vi "SVFA Real and Imaginary to Magnitude and Phase (1 Ch).vi"(0 "real spectrum":cluster{"x0":dbl, "dx":dbl, "real part":dbl[]}, 2 "imaginary spectrum":T8, 4 "spectrum info in":T2={"channel name"="", "description"="", "x-axis units"=0, "spectral info"={"spectrum type"=enum."Power [Magnitude^2]", "linear/dB"=enum."linear", "window"=0, "window size"=0, "FFT size"=0}, "engineering units"=0, "custom label"="", "dB reference [EU]"=0.0, "peak units"=enum."rms", "weighting filter"=0, "spectral density?"=FALSE, "unit label"="", "spectrum skewed?"=FALSE, "complimentary spectrum units"=enum."none"} {"x-axis units" items=["Time (s)"=0, "Frequency-CB (Hz)"=1, "Frequency-CPB (Hz)"=1248, "Frequency-Arbitrary (Hz)"=2357, "Quefrency (s)"=2, "Revolutions (rev)"=3, "Order"=4, "Speed (RPM)"=11, "Speed (rad/s)"=21, "Index"=65535]; "weighting filter" items=["Linear", "A-weighting", "B-weighting", "C-weighting", "ITU-R 468-4", "Dolby", "CCITT", "C-message", "Wb", "Wc", "Wd", "We", "Wf", "Wh", "Wj", "Wk", "Wm", "AES17 20 kHz lowpass", "AES17 40 kHz lowpass", "AES17 20 kHz highpass", "AES17 40 kHz highpass"]; "dB reference [EU]" format="%.2f"; "engineering units" items=["custom..."=0, "V"=1, "A"=21, "C"=30, "pC"=31, "s"=32, "-"=29, "Pa"=2, "N"=20, "g"=3, "m/s^2"=4, "m/s"=5, "m"=6, "mm/s"=12, "mm"=13, "micron/s"=14, "micron"=15, "in/s^2"=7, "in/s"=8, "in"=9, "mil/s"=10, "mil"=11, "rad/s^2"=16, "rad/s"=17, "rad"=18, "deg/s^2"=26, "deg/s"=27, "deg"=28, "RPM"=22, "cycle/s^2"=23, "Hz"=24, "cycle"=25, "strain"=19]; "spectral info"."window" items=["None "=0, "Hanning"=1, "Hamming"=2, "Blackman-Harris"=3, "Exact Blackman"=4, "Blackman"=5, "Flat Top"=6, "4 Term B-Harris "=7, "7 Term B-Harris"=8, "Low Sidelobe"=9, "Force - Exponential"=10, "Gaussian"=62]}, 5 "error in (no error)":errorcluster, 6 "view":T1={"dB On (F)"=FALSE, "unwrap phase (F)"=FALSE, "convert to degree (T)"=TRUE}) -> (14 "magnitude spectrum":cluster{"x0":dbl, "dx":dbl, "magnitude":dbl[]}, 15 "magnitude unit label":string, 16 "phase spectrum":cluster{"x0":dbl, "dx":dbl, "phase":dbl[]}, 17 "phase unit label":string, 18 "spectrum info out":T2={"channel name"="", "description"="", "x-axis units"=0, "spectral info"={"spectrum type"=enum."Power [Magnitude^2]", "linear/dB"=enum."linear", "window"=0, "window size"=0, "FFT size"=0}, "engineering units"=1, "custom label"="", "dB reference [EU]"=0.0, "peak units"=enum."rms", "weighting filter"=0, "spectral density?"=FALSE, "unit label"="", "spectrum skewed?"=FALSE, "complimentary spectrum units"=enum."none"} {"x-axis units" items=["Time (s)"=0, "Frequency-CB (Hz)"=1, "Frequency-CPB (Hz)"=1248, "Frequency-Arbitrary (Hz)"=2357, "Quefrency (s)"=2, "Revolutions (rev)"=3, "Order"=4, "Speed (RPM)"=11, "Speed (rad/s)"=21, "Index"=65535]; "weighting filter" items=["Linear", "A-weighting", "B-weighting", "C-weighting", "ITU-R 468-4", "Dolby", "CCITT", "C-message", "Wb", "Wc", "Wd", "We", "Wf", "Wh", "Wj", "Wk", "Wm", "AES17 20 kHz lowpass", "AES17 40 kHz lowpass", "AES17 20 kHz highpass", "AES17 40 kHz highpass"]; "dB reference [EU]" format="%.2f"; "engineering units" items=["custom..."=0, "V"=1, "A"=21, "C"=30, "pC"=31, "s"=32, "-"=29, "Pa"=2, "N"=20, "g"=3, "m/s^2"=4, "m/s"=5, "m"=6, "mm/s"=12, "mm"=13, "micron/s"=14, "micron"=15, "in/s^2"=7, "in/s"=8, "in"=9, "mil/s"=10, "mil"=11, "rad/s^2"=16, "rad/s"=17, "rad"=18, "deg/s^2"=26, "deg/s"=27, "deg"=28, "RPM"=22, "cycle/s^2"=23, "Hz"=24, "cycle"=25, "strain"=19]; "spectral info"."window" items=["None "=0, "Hanning"=1, "Hamming"=2, "Blackman-Harris"=3, "Exact Blackman"=4, "Blackman"=5, "Flat Top"=6, "4 Term B-Harris "=7, "7 Term B-Harris"=8, "Low Sidelobe"=9, "Force - Exponential"=10, "Gaussian"=62]}, 19 "error out":errorcluster)   [LabVIEW 2017]
doc: "Converts spectra from rectangular components to polar components. You can display magnitude and phase information on graphs and send this information to other Spectrum Extended Measurements VIs. Wire data to the <B>real spectrum</B> and <B>imaginary spectrum</B> inputs to determine the polymorphic instance to use or manually select the instance."
uses:
  <vilib>/addons/_NISVFA/_Shared subVIs/Controls/svc_Spectrum Info.ctl
  <vilib>/addons/_NISVFA/_Shared subVIs/Controls/svc_X-Axis Units.ctl
  <vilib>/addons/_NISVFA/_Shared subVIs/Controls/svc_Spectrum Type.ctl
  <vilib>/addons/_NISVFA/_Shared subVIs/Controls/svc_Engineering Units Text Ring.ctl
  <vilib>/addons/_NISVFA/_Shared subVIs/Controls/svc_Weighting Filter Text Ring.ctl
  <vilib>/addons/_NISVFA/_Shared subVIs/Controls/svc_Complimentary Spectrum Units.ctl
  <vilib>/addons/_NISVFA/_Shared subVIs/Common/svc_Get Weighting Enum and Labels.vi
  <vilib>/addons/_NISVFA/_Shared subVIs/Common/svc_Unit Label Lexical Class.vi
  <vilib>/addons/_NISVFA/_Shared subVIs/Common/svc_Engineering Units to Unit Label.vi
  <vilib>/addons/_NISVFA/_Shared subVIs/Common/svc_Format Value (DBL).vi
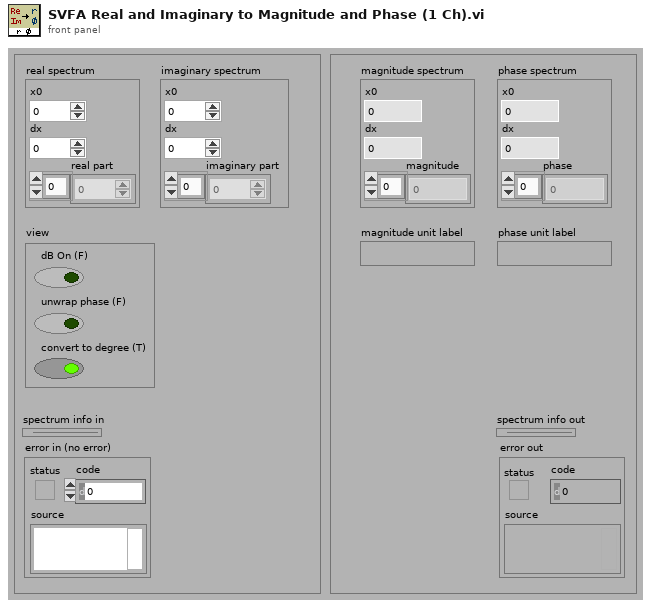
[diagram p1: front panel]
types:
  T1 = cluster{"dB On (F)":bool, "unwrap phase (F)":bool, "convert to degree (T)":bool}
  T2 = typedef "svc_Spectrum Info.ctl" = cluster{"channel name":string, "description":string, "x-axis units":T3, "spectral info":cluster{"spectrum type":T4, "linear/dB":enum16{"linear", "dB"}, "window":u16, "window size":i32, "FFT size":i32}, "engineering units":T5, "custom label":string, "dB reference [EU]":dbl, "peak units":enum16{"rms", "peak", "peak-peak"}, "weighting filter":T6, "spectral density?":bool, "unit label":string, "spectrum skewed?":bool, "complimentary spectrum units":T7}
  T3 = typedef "svc_X-Axis Units.ctl" = u16
  T4 = typedef "svc_Spectrum Type.ctl" = enum16{"FFT Spectrum [complex]", "Amplitude [Magnitude]", "Power [Magnitude^2]", "Cross Spectrum [complex]", "Frequency Response [Complex]"}
  T5 = typedef "svc_Engineering Units Text Ring.ctl" = u16
  T6 = typedef "svc_Weighting Filter Text Ring.ctl" = u16
  T7 = typedef "svc_Complimentary Spectrum Units.ctl" = enum16{"none", "radians", "degrees", "cycles", "imaginary"}
  T8 = cluster{"x0":dbl, "dx":dbl, "imaginary part":dbl[]}
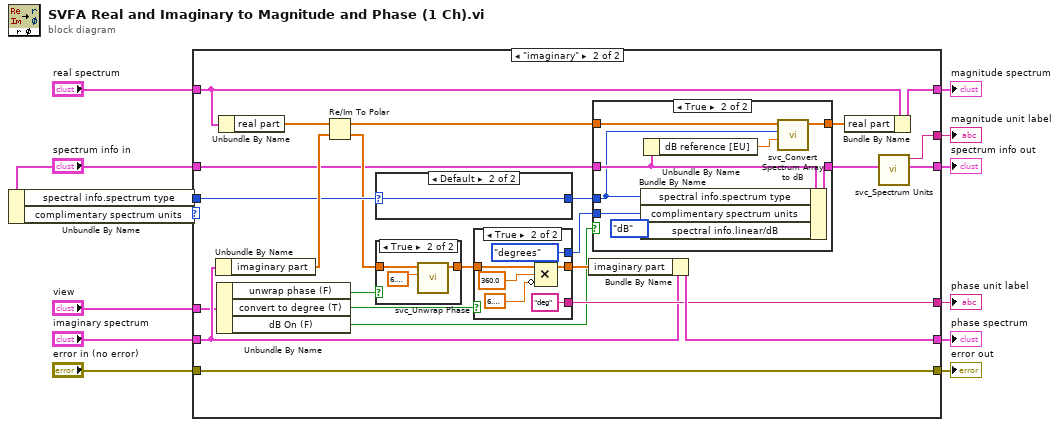
[diagram p0: block diagram]
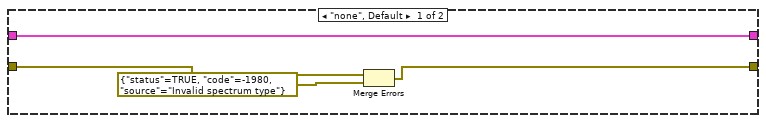
[diagram p2: hidden frame]
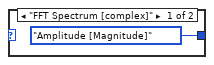
[diagram p3: hidden frame]
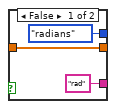
[diagram p5: hidden frame]
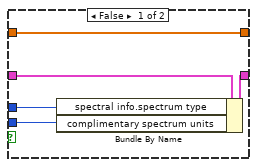
[diagram p6: hidden frame]
diagram:
  n1 = Unbundle By Name("spectrum info in") -> ("spectral info.spectrum type"=w2:T4, "complimentary spectrum units"=w5:T7)
  n2 = case shown="\"imaginary\"" w5 {
    tunnel: "real spectrum" -> [_ w39]
    tunnel: "imaginary spectrum" -> [w15 w23]
    tunnel: [_ w26] -> w11
    tunnel: "error in (no error)" -> [w17 w31]
    tunnel: [w16 w31] -> w9
    tunnel: [w15 w25] -> w8
    tunnel: [_ w20] -> w7
    tunnel: "spectrum info in" -> [_ w27]
    tunnel: w2 -> [_ w30]
    tunnel: "view" -> [_ w22]
    tunnel: [_ w24] -> w3
    tunnel: [_ w18] -> w1
    frame "none", Default {
      n3 = Merge Errors(w17, errorcluster {"status"=TRUE, "code"=-1980, "source"="Invalid spectrum type"} ("error in (no error)")) -> (w16:errorcluster)
    }
    frame "imaginary" {
      n4 = Unbundle By Name(w23) -> ("imaginary part"=w40:dbl[])
      n5 = Unbundle By Name(w22) -> ("unwrap phase (F)"=w38:bool, "convert to degree (T)"=w37:bool, "dB On (F)"=w21:bool)
      n6 = Unbundle By Name(w39) -> ("real part"=w41:dbl[])
      n7 = Re/Im To Polar(2:w40, 3:w41) -> (0:w29:dbl[], 1:w33:dbl[])
      n8 = case shown="Default" w30 {
        selector: w30 -> [_ w43]
        tunnel: [svc_Spectrum_Type."Amplitude [Magnitude]" ("spectrum type") w43] -> w36
        frame "FFT Spectrum [complex]" {
        }
        frame Default {
        }
      }
      n9 = case shown="True" w38 {
        tunnel: w29 -> [w44 w47]
        tunnel: [w44 w46] -> w34
        frame False {
        }
        frame True {
          n10 = call <vilib>:"svc_Unwrap Phase.vi"("full cycle (2pi)"=6.283185307179586 ("x"), "phase in"=w47) -> ("phase out"=w46:dbl[])  [unwired: 8 in, 1 out]
        }
      }
      n11 = case shown="True" w37 {
        tunnel: [w50 w56] -> w28
        tunnel: w34 -> [w50 w52]
        tunnel: ["rad" ("unit label (phase)") "deg" ("unit label (phase)")] -> w24
        tunnel: [svc_Complimentary_Spectrum_Units."radians" ("complimentary spectrum units") svc_Complimentary_Spectrum_Units."degrees" ("complimentary spectrum units")] -> w35
        frame False {
        }
        frame True {
          n12 = Compound Arithmetic op=MULTIPLY(w52, 360.0 ("x"), invert 6.283185307179586 ("Pi Multiplied By 2")) -> (w56:dbl[])
        }
      }
      n13 = Bundle By Name(cluster=w23, "imaginary part"=w28) -> (w25:T8)
      n14 = case shown="True" w21 {
        tunnel: w27 -> [w60 w68]
        tunnel: [w59 w69] -> w19
        tunnel: w33 -> [w61 w66]
        tunnel: [w61 w65] -> w32
        tunnel: w36 -> [w58 w64]
        tunnel: w35 -> [w57 w62]
        frame False {
          n15 = Bundle By Name(cluster=w60, "spectral info.spectrum type"=w58, "complimentary spectrum units"=w57) -> (w59:T2)
        }
        frame True {
          n16 = Bundle By Name(cluster=w68, "spectral info.spectrum type"=w64, "complimentary spectrum units"=w62, "spectral info.linear/dB"=enum16{"linear", "dB"}."dB" ("Spectral Info.linear/dB")) -> (w69:T2)
          n17 = Unbundle By Name(w68) -> ("dB reference [EU]"=w67:dbl)
          n18 = call <vilib>:"svc_Convert Spectrum Array to dB.vi"("dB reference"=w67, "spectrum type"=w64, "spectrum"=w66) -> ("spectrum in dB"=w65:dbl[])  [unwired: 8 in]
        }
      }
      n19 = Bundle By Name(cluster=w39, "real part"=w32) -> (w26:cluster{"x0":dbl, "dx":dbl, "real part":dbl[]})
      n20 = call <vilib>:"svc_Spectrum Units.vi"("spectrum info in"=w19) -> ("spectrum info out"=w20:T2, "unit label"=w18:string)  [unwired: 3 in, 2 out]
    }
  }
  "magnitude spectrum" <- w11
  "phase spectrum" <- w8
  "error out" <- w9
  "spectrum info out" <- w7
  "magnitude unit label" <- w1
  "phase unit label" <- w3
